vi "Initialize Incoming.vi"(8 "error in (no error)":errorcluster, 10 "OnCompile Variables":T12={"Name"="", "XNET Settings"={"Database"="", "Cluster"="", "Port"="", "Baud rate [Bd]"=500000, "Termination"=1, "CAN I/O Mode"=0, "FD Baud rate [Bd]"=500000, "Priority"=100, "Use Legacy"=FALSE, "FD ISO Mode"=0}, "Frames"=[], "986x Support"={"Enable"=FALSE, "RIO Device"="", "Bitfile"=path ""}, "Incoming Signal Info"={"Signal Settings Out"=[], "Signal_Valid_Values"=[], "Signal Names"=[], "ProtCtrValues"=[], "AllSigValues"=[]}, "Incoming Frames"=[]} {"Incoming Frames"."Protection Configurations"."CRC Channels"."Data Type" items=["Signed", "Unsigned", "IEEE Float"]; "Incoming Signal Info"."Signal Settings Out"."Protection Configuration"."CRC Channels"."Data Type" items=["Signed", "Unsigned", "IEEE Float"]; "XNET Settings"."FD ISO Mode" items=["ISO", "Non ISO", "ISO Legacy"]; "XNET Settings"."CAN I/O Mode" items=["CAN 2.0", "CAN FD", "CAN FD+BRS"]; "XNET Settings"."Termination" items=["Off", "On"]; "Frames"."Protection Configurations"."CRC Channels"."Data Type" items=["Signed", "Unsigned", "IEEE Float"]}, 11 "RT Configuration In":T1={"Name"="", "Priority"=100, "CAN Session"="", "Frame Count"=0, "Frames"=[], "FPGA Session"=0, "XNET Settings"={"Database"="", "Cluster"="", "Port"="", "Baud rate [Bd]"=0, "Termination"=0, "CAN I/O Mode"=0, "FD Baud rate [Bd]"=500000, "Priority"=100, "Use Legacy"=FALSE, "FD ISO Mode"=0}, "Incoming Frame Session"="", "Incoming Session Invalid"=FALSE, "Incoming Signal Info"={"Signal_Valid_Values"=[], "Signal Names"=[], "Signal Settings Out"=[], "Frame Receive Time Values"=[], "ProtCtr Sig Values"=[], "All Sig Values"=[]}, "Signal Values"=[]} {"Incoming Signal Info"."Signal Settings Out"."Protection Configuration"."CRC Channels"."Data Type" items=["Signed", "Unsigned", "IEEE Float"]; "XNET Settings"."FD ISO Mode" items=["ISO", "Non ISO", "ISO Legacy"]; "XNET Settings"."CAN I/O Mode" items=["CAN 2.0", "CAN FD", "CAN FD+BRS"]; "XNET Settings"."Termination" items=["Off", "On"]; "Frames"."Protection Configurations"."CRC Channels"."Data Type" items=["Signed", "Unsigned", "IEEE Float"]}) -> (0 "error out":errorcluster, 3 "RT Configuration Out":T1={"Name"="", "Priority"=100, "CAN Session"="", "Frame Count"=0, "Frames"=[], "FPGA Session"=0, "XNET Settings"={"Database"="", "Cluster"="", "Port"="", "Baud rate [Bd]"=0, "Termination"=0, "CAN I/O Mode"=0, "FD Baud rate [Bd]"=500000, "Priority"=100, "Use Legacy"=FALSE, "FD ISO Mode"=0}, "Incoming Frame Session"="", "Incoming Session Invalid"=FALSE, "Incoming Signal Info"={"Signal_Valid_Values"=[], "Signal Names"=[], "Signal Settings Out"=[], "Frame Receive Time Values"=[], "ProtCtr Sig Values"=[], "All Sig Values"=[]}, "Signal Values"=[]} {"Incoming Signal Info"."Signal Settings Out"."Protection Configuration"."CRC Channels"."Data Type" items=["Signed", "Unsigned", "IEEE Float"]; "XNET Settings"."FD ISO Mode" items=["ISO", "Non ISO", "ISO Legacy"]; "XNET Settings"."CAN I/O Mode" items=["CAN 2.0", "CAN FD", "CAN FD+BRS"]; "XNET Settings"."Termination" items=["Off", "On"]; "Frames"."Protection Configurations"."CRC Channels"."Data Type" items=["Signed", "Unsigned", "IEEE Float"]})   [LabVIEW 2019]
uses:
  Addon Shared/Types/Exported.OnCompile.ctl
  Addon Shared/Types/XNET Settings.ctl
  SubModules/Frame-Protection-Support/Source/Shared/Types/Exported Frame Settings.ctl
  SubModules/Frame-Protection-Support/Source/Shared/Types/Exported Frame Type.ctl
  SubModules/Frame-Protection-Support/Source/Shared/Types/Exported Protection Settings.ctl
  SubModules/Frame-Protection-Support/Source/Shared/Types/Protection Type.ctl
  SubModules/Frame-Protection-Support/Source/Shared/Types/XNET Signal Configuration.ctl
  SubModules/Frame-Protection-Support/Source/Shared/Types/Exported Counter Settings.ctl
  SubModules/Frame-Protection-Support/Source/Shared/Types/Exported Event Trigger Type.ctl
  Addon Shared/Types/986x.ctl
  SubModules/Frame-Protection-Support/Source/Shared/Types/Incoming Signal Info.ctl
  SubModules/Frame-Protection-Support/Source/Shared/Types/Exported Signal Settings.ctl
  Types/RT Async Engine Settings.ctl
  SubModules/Frame-Protection-Support/Source/Engine/Types/RT Frame Settings.ctl
  SubModules/Frame-Protection-Support/Source/Engine/Types/RT Protection Configuration.ctl
  SubModules/Frame-Protection-Support/Source/Shared/Types/RT_Incoming_Signal_Info.ctl
  SubModules/Frame-Protection-Support/Source/Shared/Types/RT Exported Signal Settings.ctl
  <vilib>/xnet/xnet.llb/XNET Create Session (Signal Input XY).vi
  <resource>/objmgr/xnet.rc
  SubModules/Frame-Protection-Support/Source/Shared/Protection and Counter Support Shared.lvlib
  Addon Shared/Protection and Counter Addon Shared.lvlib
  SubModules/Frame-Protection-Support/Source/Engine/Protection and Counter Support Engine.lvlib
  Protection and Counter Addon Engine.lvlib
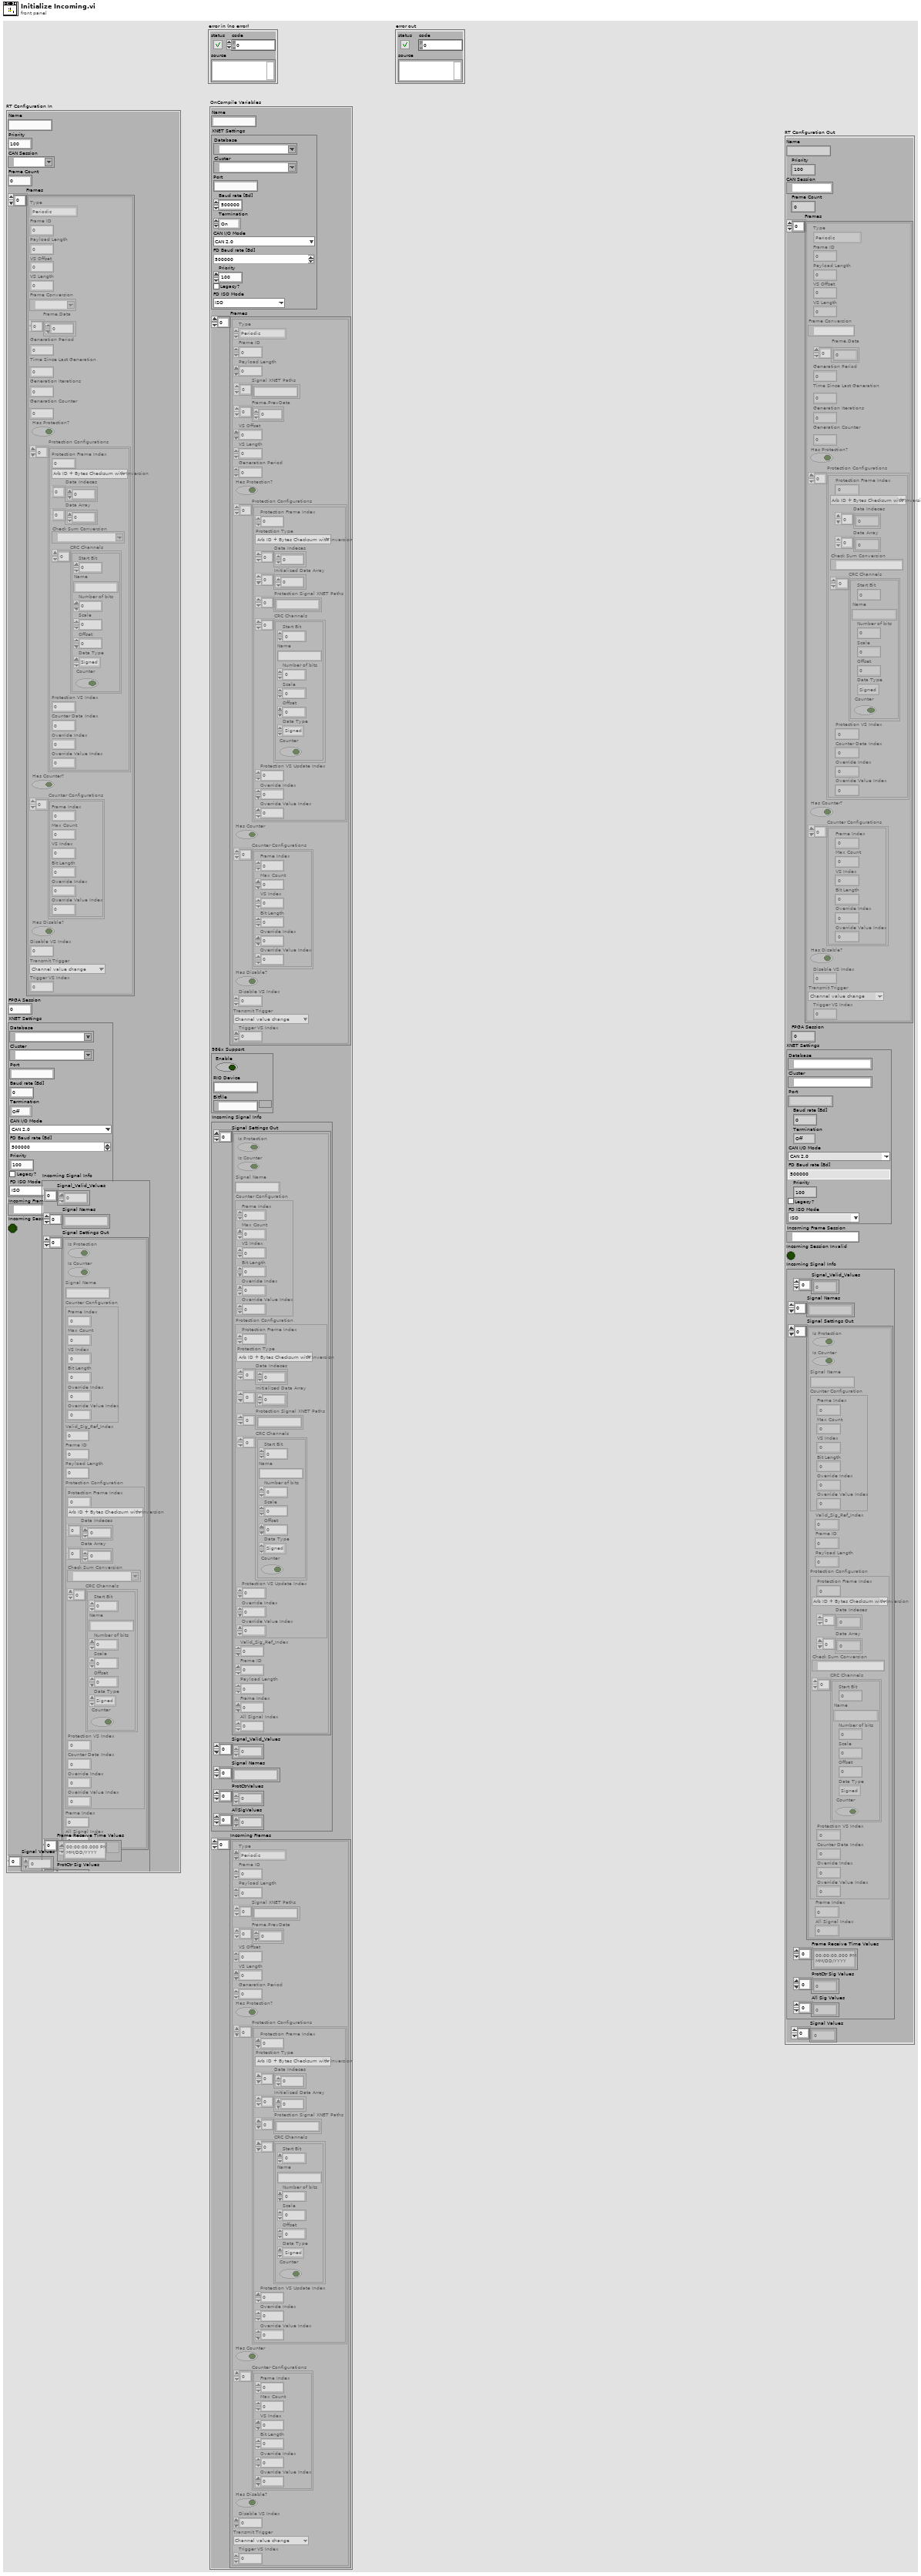
[diagram p1: front panel]
types:
  T1 = typedef "Protection and Counter Addon Engine.lvlib/RT Async Engine Settings.ctl" = cluster{"Name":string, "Priority":i32, "CAN Session":refnum<k21>, "Frame Count":i32, "Frames":T2[], "FPGA Session":u32, "XNET Settings":T9, "Incoming Frame Session":refnum<k21>, "Incoming Session Invalid":bool, "Incoming Signal Info":T10, "Signal Values":dbl[]}
  T2 = typedef "Protection and Counter Support Engine.lvlib/RT Frame Settings.ctl" = cluster{"Type":T3, "Frame ID":u32, "Payload Length":u32, "VS Offset":i32, "VS Length":i32, "Frame Conversion":refnum<k21>, "Frame.Data":dbl[], "Generation Period":u32, "Time Since Last Generation":u32, "Generation Iterations":u32, "Generation Counter":u32, "Has Protection?":bool, "Protection Configurations":T4[], "Has Counter?":bool, "Counter Configurations":T7[], "Has Disable?":bool, "Disable VS Index":i32, "Transmit Trigger":T8, "Trigger VS Index":i32}
  T3 = typedef "Protection and Counter Support Shared.lvlib/Exported Frame Type.ctl" = enum16{"Periodic", "Event", "Periodic/Event"}
  T4 = typedef "Protection and Counter Support Engine.lvlib/RT Protection Configuration.ctl" = cluster{"Protection Frame Index":i32, "Protection Type":T5, "Data Indeces":i32[], "Data Array":dbl[], "Check Sum Conversion":refnum<k21>, "CRC Channels":T6[], "Protection VS Index":i32, "Counter Data Index":i32, "Override Index":i32, "Override Value Index":i32}
  T5 = typedef "Protection and Counter Support Shared.lvlib/Protection Type.ctl" = enum16{"Arb ID + Bytes Checksum with Inversion", "Arb ID + Bytes CRC with Inversion", "Reversed Raw Signal Checksum with Inversion", "Concatenated Two's Compliment"}
  T6 = typedef "Protection and Counter Support Shared.lvlib/XNET Signal Configuration.ctl" = cluster{"Start Bit":i32, "Name":string, "Number of bits":i32, "Scale":dbl, "Offset":dbl, "Data Type":u32, "Counter":bool}
  T7 = typedef "Protection and Counter Support Shared.lvlib/Exported Counter Settings.ctl" = cluster{"Frame Index":i32, "Max Count":dbl, "VS Index":i32, "Bit Length":i64, "Override Index":i32, "Override Value Index":i32}
  T8 = typedef "Protection and Counter Support Shared.lvlib/Exported Event Trigger Type.ctl" = enum16{"Channel value change", "Trigger channel (not zero)", "Channel value change or trigger channel (not zero)", "Trigger channel (any value change)", "Channel value change or trigger channel (any value change)"}
  T9 = typedef "Protection and Counter Addon Shared.lvlib/XNET Settings.ctl" = cluster{"Database":refnum<k21>, "Cluster":refnum<k21>, "Port":string, "Baud rate [Bd]":u64, "Termination":u32, "CAN I/O Mode":u32, "FD Baud rate [Bd]":u64, "Priority":i32, "Use Legacy":bool, "FD ISO Mode":u32}
  T10 = typedef "RT_Incoming_Signal_Info.ctl" = cluster{"Signal_Valid_Values":dbl[], "Signal Names":string[], "Signal Settings Out":T11[], "Frame Receive Time Values":timestamp[], "ProtCtr Sig Values":dbl[], "All Sig Values":dbl[]}
  T11 = typedef "RT Exported Signal Settings.ctl" = cluster{"Is Protection":bool, "Is Counter":bool, "Signal Name":string, "Counter Configuration":T7, "Valid_Sig_Ref_Index":i32, "Frame ID":u32, "Payload Length":u32, "Protection Configuration":T4, "Frame Index":i32, "All Signal Index":i32}
  T12 = typedef "Protection and Counter Addon Shared.lvlib/Exported.OnCompile.ctl" = cluster{"Name":string, "XNET Settings":T9, "Frames":T13[], "986x Support":T15, "Incoming Signal Info":T16, "Incoming Frames":T13[]}
  T13 = typedef "Protection and Counter Support Shared.lvlib/Exported Frame Settings.ctl" = cluster{"Type":T3, "Frame ID":u32, "Payload Length":u32, "Signal XNET Paths":string[], "Frame.PrevData":dbl[], "VS Offset":i32, "VS Length":i32, "Generation Period":u32, "Has Protection?":bool, "Protection Configurations":T14[], "Has Counter":bool, "Counter Configurations":T7[], "Has Disable?":bool, "Disable VS Index":i32, "Transmit Trigger":T8, "Trigger VS Index":i32}
  T14 = typedef "Protection and Counter Support Shared.lvlib/Exported Protection Settings.ctl" = cluster{"Protection Frame Index":i32, "Protection Type":T5, "Data Indeces":i32[], "Initialized Data Array":dbl[], "Protection Signal XNET Paths":string[], "CRC Channels":T6[], "Protection VS Update Index":i32, "Override Index":i32, "Override Value Index":i32}
  T15 = typedef "Protection and Counter Addon Shared.lvlib/986x.ctl" = cluster{"Enable":bool, "RIO Device":string, "Bitfile":path}
  T16 = typedef "Incoming Signal Info.ctl" = cluster{"Signal Settings Out":T17[], "Signal_Valid_Values":dbl[], "Signal Names":string[], "ProtCtrValues":dbl[], "AllSigValues":dbl[]}
  T17 = typedef "Exported Signal Settings.ctl" = cluster{"Is Protection":bool, "Is Counter":bool, "Signal Name":string, "Counter Configuration":T7, "Protection Configuration":T14, "Valid_Sig_Ref_Index":i32, "Frame ID":u32, "Payload Length":u32, "Frame Index":i32, "All Signal Index":i32}
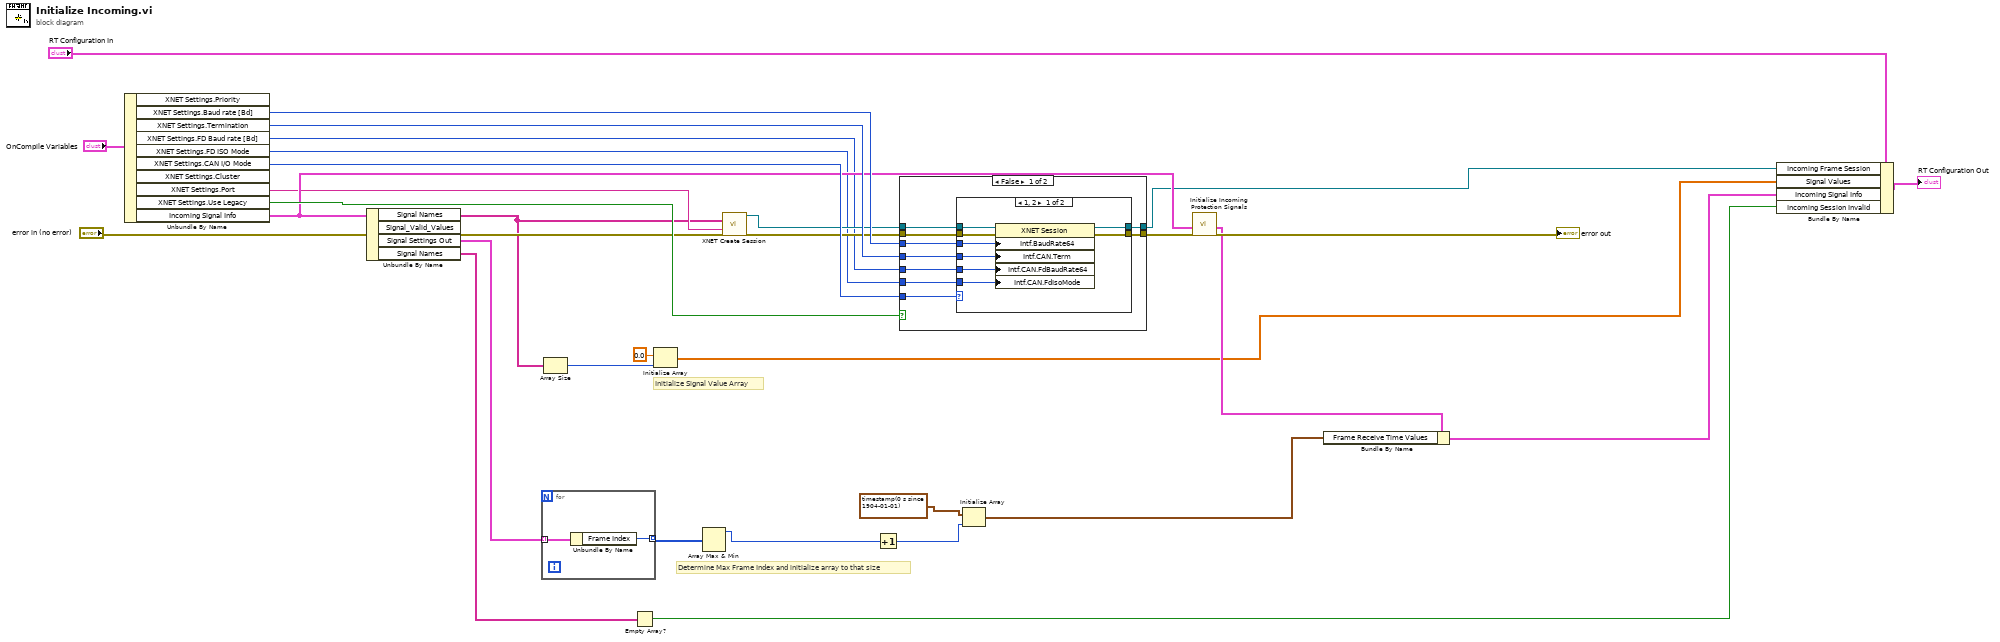
[diagram p0: block diagram]
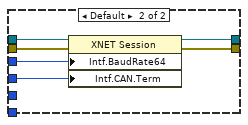
[diagram p2: hidden frame]
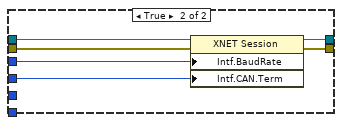
[diagram p3: hidden frame]
diagram:
  # "Determine Max Frame Index and initialize array to that size"
  # "Initialize Signal Value Array"
  n1 = Unbundle By Name("OnCompile Variables") -> ("XNET Settings.Baud rate [Bd]"=w28:u64, "XNET Settings.Termination"=w29:u32, "XNET Settings.FD Baud rate [Bd]"=w2:u64, "XNET Settings.FD ISO Mode"=w1:u32, "XNET Settings.CAN I/O Mode"=w30:u32, "XNET Settings.Port"=w12:string, "XNET Settings.Use Legacy"=w27:bool, "Incoming Signal Info"=w21:T16)  [unwired: 2 out]
  n2 = Unbundle By Name(w21) -> ("Signal Names"=w11:string[], "Signal Settings Out"=w20:T17[], "Signal Names"=w5:string[])  [unwired: 1 out]
  n3 = for {
    tunnel: w20 -> [w33] mode=indexing
    tunnel: [w32] -> w18 mode=indexing
    n4 = Unbundle By Name(w33) -> ("Frame Index"=w32:i32)
  }
  n5 = Array Size(array=w11) -> (size(s)=w26:i32)
  n6 = Empty Array?(array=w5) -> (empty?=w4:bool)
  n7 = Initialize Array(0.0 ("element"), w26) -> (w6:dbl[])
  n8 = Array Max & Min(array=w18) -> (max value=w17:i32)  [unwired: 3 out]
  n9 = call-poly <vilib>:"XNET Create Session.vi"("signal list"=w11, "interface"=w12, "error in (no error)"="error in (no error)") -> ("session out"=w10:refnum<k21>, "error out"=w13:errorcluster)  [unwired: 11 in]
  n10 = Increment(x=w17) -> (x+1=w19:i32)
  n11 = case shown="False" w27 {
    tunnel: w13 -> [w42 w62]
    tunnel: w10 -> [w41 w61]
    tunnel: [w40 w60] -> w24
    tunnel: w30 -> [w36 _]
    tunnel: w29 -> [w39 w57]
    tunnel: w28 -> [w38 w58]
    tunnel: [w37 w59] -> w3
    tunnel: w2 -> [w35 _]
    tunnel: w1 -> [w34 _]
    frame False {
      n12 = case shown="1, 2" w36 {
        tunnel: w42 -> [w50 w56]
        tunnel: w41 -> [w49 w55]
        tunnel: [w48 w54] -> w40
        tunnel: w39 -> [w47 w53]
        tunnel: w38 -> [w46 w52]
        tunnel: [w45 w51] -> w37
        tunnel: w35 -> [w44 _]
        tunnel: w34 -> [w43 _]
        frame 1, 2 {
          n13 = property class="XNET Session"(reference=w49, error in=w50, "Intf.BaudRate64"=w46, "Intf.CAN.Term"=w47, "Intf.CAN.FdBaudRate64"=w44, "Intf.CAN.FdIsoMode"=w43) -> (reference out=w45:refnum<k21>, error out=w48:errorcluster)
        }
        frame Default {
          n14 = property class="XNET Session"(reference=w55, error in=w56, "Intf.BaudRate64"=w52, "Intf.CAN.Term"=w53) -> (reference out=w51:refnum<k21>, error out=w54:errorcluster)
        }
      }
    }
    frame True {
      n15 = property class="XNET Session"(reference=w61, error in=w62, "Intf.BaudRate"=w58, "Intf.CAN.Term"=w57) -> (reference out=w59:refnum<k21>, error out=w60:errorcluster)
    }
  }
  n16 = Initialize Array(timestamp(0 s since 1904-01-01), w19) -> (w15:timestamp[])
  n17 = call "Initialize Incoming Protection Signals.vi"("error in (no error)"=w24, "Incoming Signal Info In"=w21) -> ("error out"=→"error out":errorcluster, "RT Incoming Signal Info"=w16:T10)  [unwired: 8 in]
  n18 = Bundle By Name(cluster=w16, "Frame Receive Time Values"=w15) -> (w8:T10)
  n19 = Bundle By Name(cluster="RT Configuration In", "Incoming Frame Session"=w3, "Signal Values"=w6, "Incoming Signal Info"=w8, "Incoming Session Invalid"=w4) -> (→"RT Configuration Out":T1)
